vi "FTW-STR-Array-Delimit.vi"(5 "Array of Strings":string[](array[string]), 7 "Delimiter":string=",") -> (6 "Delimited String":string)   [LabVIEW 2015]
panel:
  # "Inputs"
  # "Outputs"
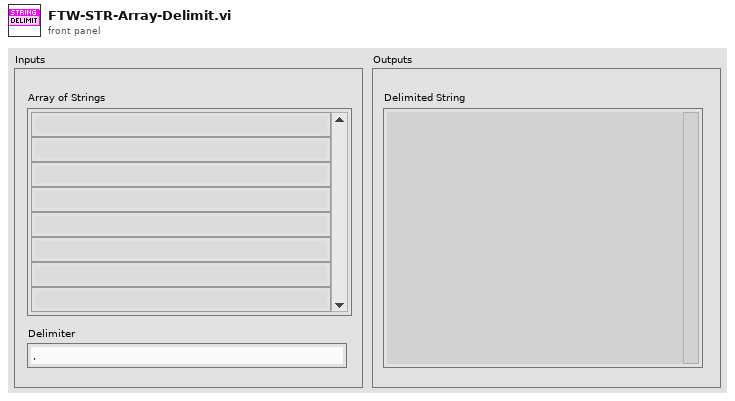
[diagram p1: front panel]
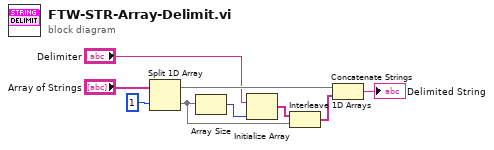
[diagram p0: block diagram]
diagram:
  n1 = Split 1D Array(array="Array of Strings", index=1) -> (first subarray=w7:string[], second subarray=w2:string[])
  n2 = Array Size(array=w2) -> (size(s)=w5:i32)
  n3 = Initialize Array("Delimiter", w5) -> (w3:string[])
  n4 = Interleave 1D Arrays(w3, w2) -> (w1:string[])
  n5 = Concatenate Strings(w7, w1) -> (→"Delimited String":string)
